vi "process.vi"(8 "error in":errorcluster, 9 "result allocation":T1, 10 "parameters":T1, 11 "AppStateMachine runtime in":refnum<class "AppStateMachine runtime.lvclass">) -> (0 "error out":errorcluster, 1 "results":T1, 2 "parameter allocation":T1, 3 "AppStateMachine runtime out":refnum<class "AppStateMachine runtime.lvclass">)   [LabVIEW 2017, in "AppStateMachine runtime.lvclass"]
doc: "Provides an interface for information processing by a module at runtime. While this interface performs no operations, a child should provide an override which may process data in any manner necessary."
uses:
  AppStateMachine runtime.lvclass
  <vilib>/NI/Tag Bus/table/data table.ctl
  AppStateMachine runtime.lvclass/AppStateMachine runtime.ctl
  State.ctl
  <vilib>/NI/Tag Bus/table/data table.lvlib
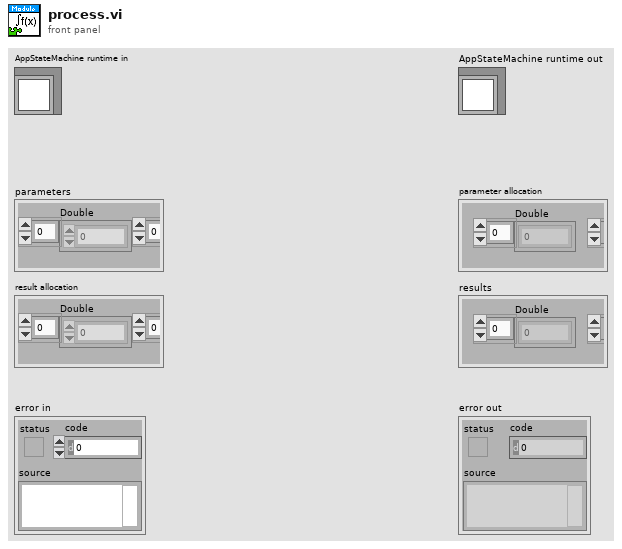
[diagram p1: front panel]
types:
  T1 = typedef "tag bus.lvlib/data table.lvlib/data table.ctl" = cluster{"Double":dbl[], "Single":sgl[], "I64":i64[], "I32":i32[], "I16":i16[], "I8":i8[], "U64":u64[], "U32":u32[], "U16":u16[], "U8":u8[], "Boolean":bool[], "String":string[], "Array of Double":cluster{"DBL Array":dbl[]}[], "Array of Single":cluster{"SGL Array":sgl[]}[], "Array of I64":cluster{"I64 Array":i64[]}[], "Array of I32":cluster{"I32 Array":i32[]}[], "Array of I16":cluster{"I16 Array":i16[]}[], "Array of I8":cluster{"I8 Array":i8[]}[], "Array of U64":cluster{"U64 Array":u64[]}[], "Array of U32":cluster{"U32 Array":u32[]}[], "Array of U16":cluster{"U16 Array":u16[]}[], "Array of U8":cluster{"U8 Array":u8[]}[], "Array of Boolean":cluster{"Boolean Array":bool[]}[], "Array of String":cluster{"String Array":string[]}[]}
  T2 = typedef "AppStateMachine runtime.lvclass/State.ctl" = enum16{"Initialize", "Idle", "Starting", "Running", "Stopping"}
  T3 = typedef "AppStateMachine configuration.lvclass/parameter data indices.ctl" = cluster{"Double.CPU":i32, "Double.Memory":i32, "Double.Disk":i32}
  T4 = typedef "AppStateMachine configuration.lvclass/result data indices.ctl" = cluster{"U16.State":i32, "String.LastCmd":i32}
  T5 = typedef "AppStateMachine runtime.lvclass/parameter user data.ctl" = cluster{"CPU":dbl, "Memory":dbl, "Disk":dbl}
  T6 = typedef "AppStateMachine runtime.lvclass/result user data.ctl" = cluster{"State":u16, "LastCmd":string}
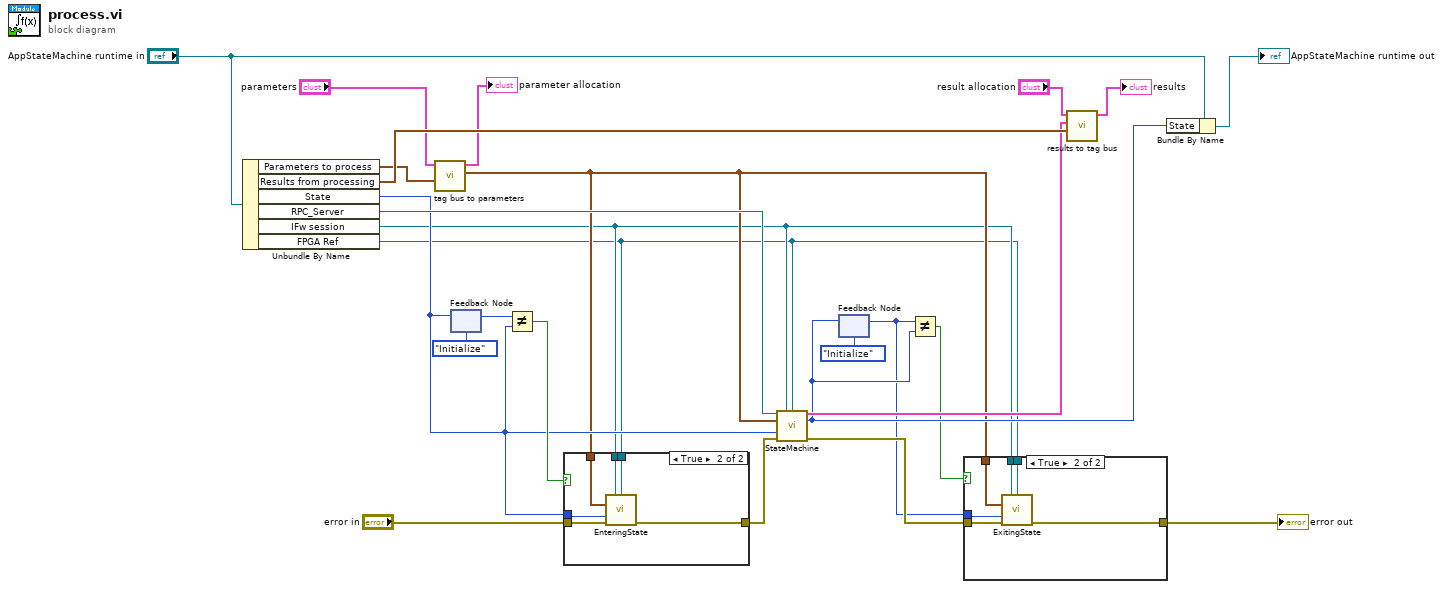
[diagram p0: block diagram]
diagram:
  n1 = Unbundle By Name("AppStateMachine runtime in") -> ("Parameters to process"=w20:T3, "Results from processing"=w23:T4, "State"=w11:T2, "RPC_Server"=w18:refnum<class "JSONRPC Server.lvclass">, "IFw session"=w4:refnum<class "niInstr FIFO Register Bus v1 Host.lvclass">, "FPGA Ref"=w3:refnum<k20>)
  n2 = call "tag bus to parameters.vi"("indices"=w20, "tag bus in"="parameters") -> ("data cluster"=w5:T5, "tag bus out"=→"parameter allocation":T1)  [unwired: 8 in]
  n3 = feedback-in #1(w11) -> ()
  n4 = feedback #1(State."Initialize" ("State")) -> (w14:T2)
  n5 = Not Equal?(x=w14, y=w11) -> (x != y?=w13:bool)
  n6 = case shown="True" w13 {
    tunnel: "error in" -> [w26 w32]
    tunnel: w11 -> [_ w30]
    tunnel: [w26 w31] -> w10
    tunnel: w5 -> [_ w29]
    tunnel: w4 -> [_ w28]
    tunnel: w3 -> [_ w27]
    frame False {
    }
    frame True {
      n7 = call "EnteringState.vi"("IFw session"=w28, "FPGA Ref"=w27, "SM inputs"=w29, "EnteringState"=w30, "error in (no error)"=w32) -> ("error out"=w31:errorcluster)  [unwired: 10 in]
    }
  }
  n8 = call "StateMachine.vi"("JSONRPC Server in"=w18, "IFw session"=w4, "FPGA Ref"=w3, "SM inputs"=w5, "State In"=w11, "error in (no error)"=w10) -> ("SM outputs"=w19:T6, "State Out"=w8:T2, "error out"=w6:errorcluster)  [unwired: 7 in]
  n9 = feedback #2(State."Initialize" ("State")) -> (w2:T2)
  n10 = feedback-in #2(w8) -> ()
  n11 = Not Equal?(x=w2, y=w8) -> (x != y?=w7:bool)
  n12 = case shown="True" w7 {
    tunnel: w6 -> [w33 w39]
    tunnel: w5 -> [_ w38]
    tunnel: w4 -> [_ w37]
    tunnel: w3 -> [_ w36]
    tunnel: w2 -> [_ w35]
    tunnel: [w33 w34] -> w1
    frame False {
    }
    frame True {
      n13 = call "ExitingState.vi"("IFw session"=w37, "FPGA Ref"=w36, "SM inputs"=w38, "ExitingState"=w35, "error in (no error)"=w39) -> ("error out"=w34:errorcluster)  [unwired: 10 in]
    }
  }
  "error out" <- w1
  n14 = call "results to tag bus.vi"("indices"=w23, "data cluster"=w19, "tag bus in"="result allocation") -> ("tag bus out"=→"results":T1)  [unwired: 8 in]
  n15 = Bundle By Name(cluster="AppStateMachine runtime in", "State"=w8) -> (→"AppStateMachine runtime out":refnum<class "AppStateMachine runtime.lvclass">)
